vi "Unicast_UDP_message.vi"(5 "message":string, 6 "error in":errorcluster, 8 "port (60434)":u16=60434, 9 "address":string="236.6.6.8") -> (0 "error out":errorcluster, 4 "response":T1)   [LabVIEW 2014, in "Raspberry Pi Compatible Compiler for LabVIEW.lvlib" / "Autodetect.lvlib"]
doc: "Broadcasts a message to the default multicast port for the devices.\n\nMulticast address = 236.6.6.8\nPort = 60434\n\nDefault message is *IDN? to return the hostname"
uses:
  Autodetect.lvlib
  TypeDefs/UDP_Response_TD.ctl
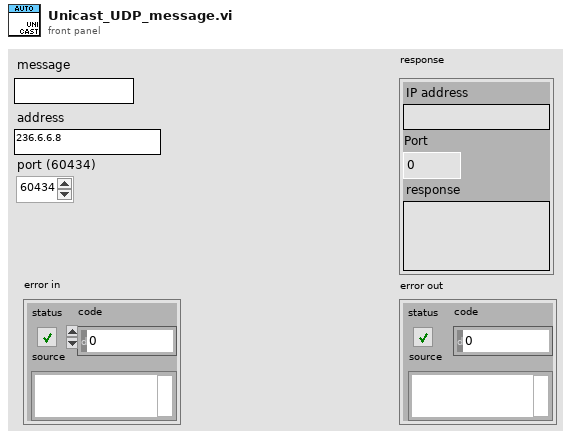
[diagram p1: front panel]
types:
  T1 = typedef "Raspberry Pi Compatible Compiler for LabVIEW.lvlib/Autodetect.lvlib/UDP_Response_TD.ctl" = cluster{"IP address":string, "Port":u16, "response":string}
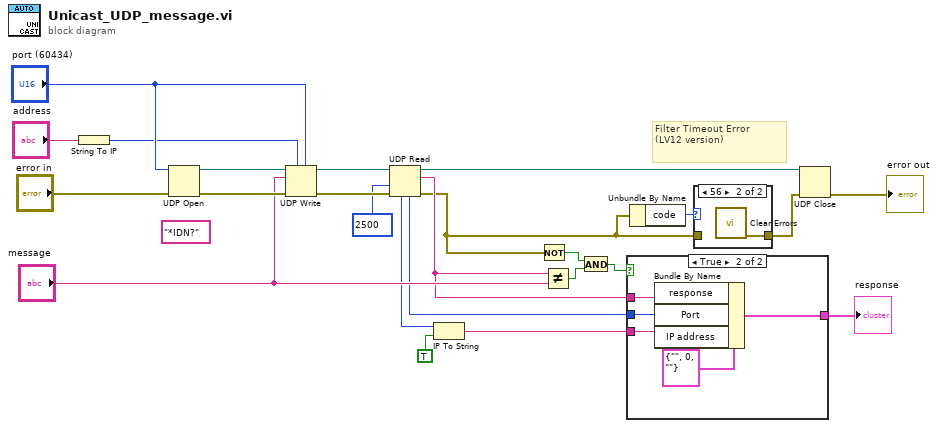
[diagram p0: block diagram]
diagram:
  (unwired) "*IDN?" ("data in")
  # "Filter Timeout Error\n(LV12 version)"
  n1 = String To IP(1:"address") -> (0:w4:u32)
  n2 = UDP Open(8:"error in", 11:"port (60434)") -> (port=w23:refnum<k16>, 0:w22:errorcluster)  [unwired: 3 in, 1 out]
  n3 = UDP Write(address=w4, port or service name="port (60434)", connection ID=w23, data in="message", 8:w22) -> (error out=w19:errorcluster, 3:w20:refnum<k16>)  [unwired: 1 in]
  n4 = UDP Read(connection ID=w20, timeout ms (25000)=2500, 8:w19) -> (data out=w9:string, error out=w1:errorcluster, 3:w18:refnum<k16>, 4:w10:u16, 6:w12:u32)  [unwired: 1 out]
  n5 = IP To String(1:TRUE ("dot notation? (F)"), 2:w12) -> (0:w11:string)
  n6 = Not(x=w1) -> (.not. x?=w7:bool)
  n7 = Not Equal?(x=w9, y="message") -> (x != y?=w8:bool)
  n8 = And(x=w7, y=w8) -> (x .and. y?=w6:bool)
  n9 = case shown="True" w6 {
    tunnel: w11 -> [_ w28]
    tunnel: w10 -> [_ w27]
    tunnel: w9 -> [_ w26]
    tunnel: [_ w25] -> w5
    frame False {
    }
    frame True {
      n10 = Bundle By Name(cluster=T1 {"IP address"="", "Port"=0, "response"=""}, "response"=w26, "Port"=w27, "IP address"=w28) -> (w25:T1)
    }
  }
  "response" <- w5
  n11 = Unbundle By Name(w1) -> ("code"=w3:i32)
  n12 = case shown="56" w3 {
    tunnel: [w30 w31] -> w2
    tunnel: w1 -> [w30 _]
    frame Default {
    }
    frame 56 {
      n13 = call <vilib>:"Clear Errors.vi"() -> ("error out"=w31:errorcluster)  [unwired: 6 in, 1 out]
    }
  }
  n14 = UDP Close(connection ID=w18, 8:w2) -> (error out=→"error out":errorcluster)  [unwired: 1 out]
